vi "uc480_SubVI_Example_GetExposure.vi"(0 ".NET (Reference)":refnum<k24>, 11 "Error In":errorcluster) -> (4 "Exposure":dbl, 6 "Inc":dbl, 8 "Min":dbl, 10 "Max":dbl, 15 "Error out":errorcluster caption="Error Out")   [LabVIEW 2016]
uses:
  C:/Users/Anatec i3/Desktop/Labview Projects/IR OPO Controller/Branches/XPS version/uc480DotNet.dll
  uc480DotNet.dll
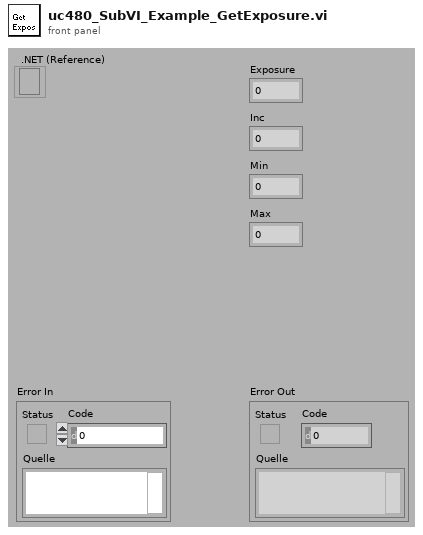
[diagram p1: front panel]
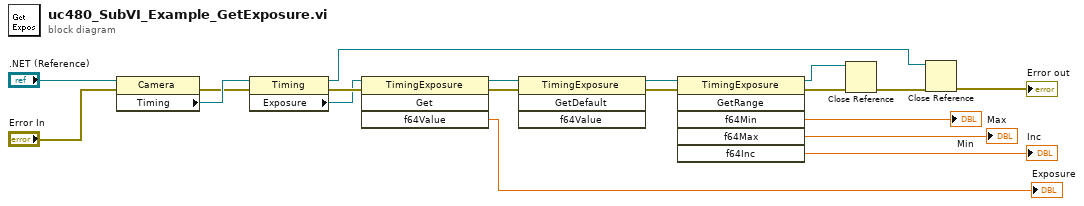
[diagram p0: block diagram]
diagram:
  n1 = property class="Camera"(reference=".NET (Reference)", error in="Error In") -> (error out=w18:errorcluster, "Timing"=w19:refnum<k24>)  [unwired: 1 out]
  n2 = property class="Timing"(reference=w19, error in=w18) -> (reference out=w1:refnum<k24>, error out=w17:errorcluster, "Exposure"=w16:refnum<k24>)
  n3 = invoke class="TimingExposure" method="Get"(reference=w16, error in=w17) -> (reference out=w15:refnum<k24>, error out=w14:errorcluster, "f64Value"=→"Exposure":dbl)  [unwired: 2 in, 1 out]
  n4 = invoke class="TimingExposure" method="GetDefault"(reference=w15, error in=w14) -> (reference out=w12:refnum<k24>, error out=w13:errorcluster)  [unwired: 2 in, 2 out]
  n5 = invoke class="TimingExposure" method="GetRange"(reference=w12, error in=w13) -> (reference out=w4:refnum<k24>, error out=w5:errorcluster, "f64Min"=→"Min":dbl, "f64Max"=→"Max":dbl, "f64Inc"=→"Inc":dbl)  [unwired: 4 in, 1 out]
  n6 = Close Reference(reference=w4, error in (no error)=w5) -> (error out=w3:errorcluster)
  n7 = Close Reference(reference=w1, error in (no error)=w3) -> (error out=→"Error out":errorcluster)
